vi "FindColllisionPoints.vi"(6 "enemy_robots":T1[](array[typedef]), 7 "our_robots":T1[](array[typedef]), 8 "Robot in":T1, 9 "Goal":dbl[](array[numeric]), 10 "Initial State":dbl[](array[numeric]), 11 "ball":dbl[](array[numeric])) -> (2 "Collision Points":dbl[][](array[numeric]))   [LabVIEW 2017]
uses:
  Core/AI Robot.ctl
  Intel/Functions Enum.ctl
  Intel/AttackerStates.ctl
  PathDests.ctl
  PathDest.ctl
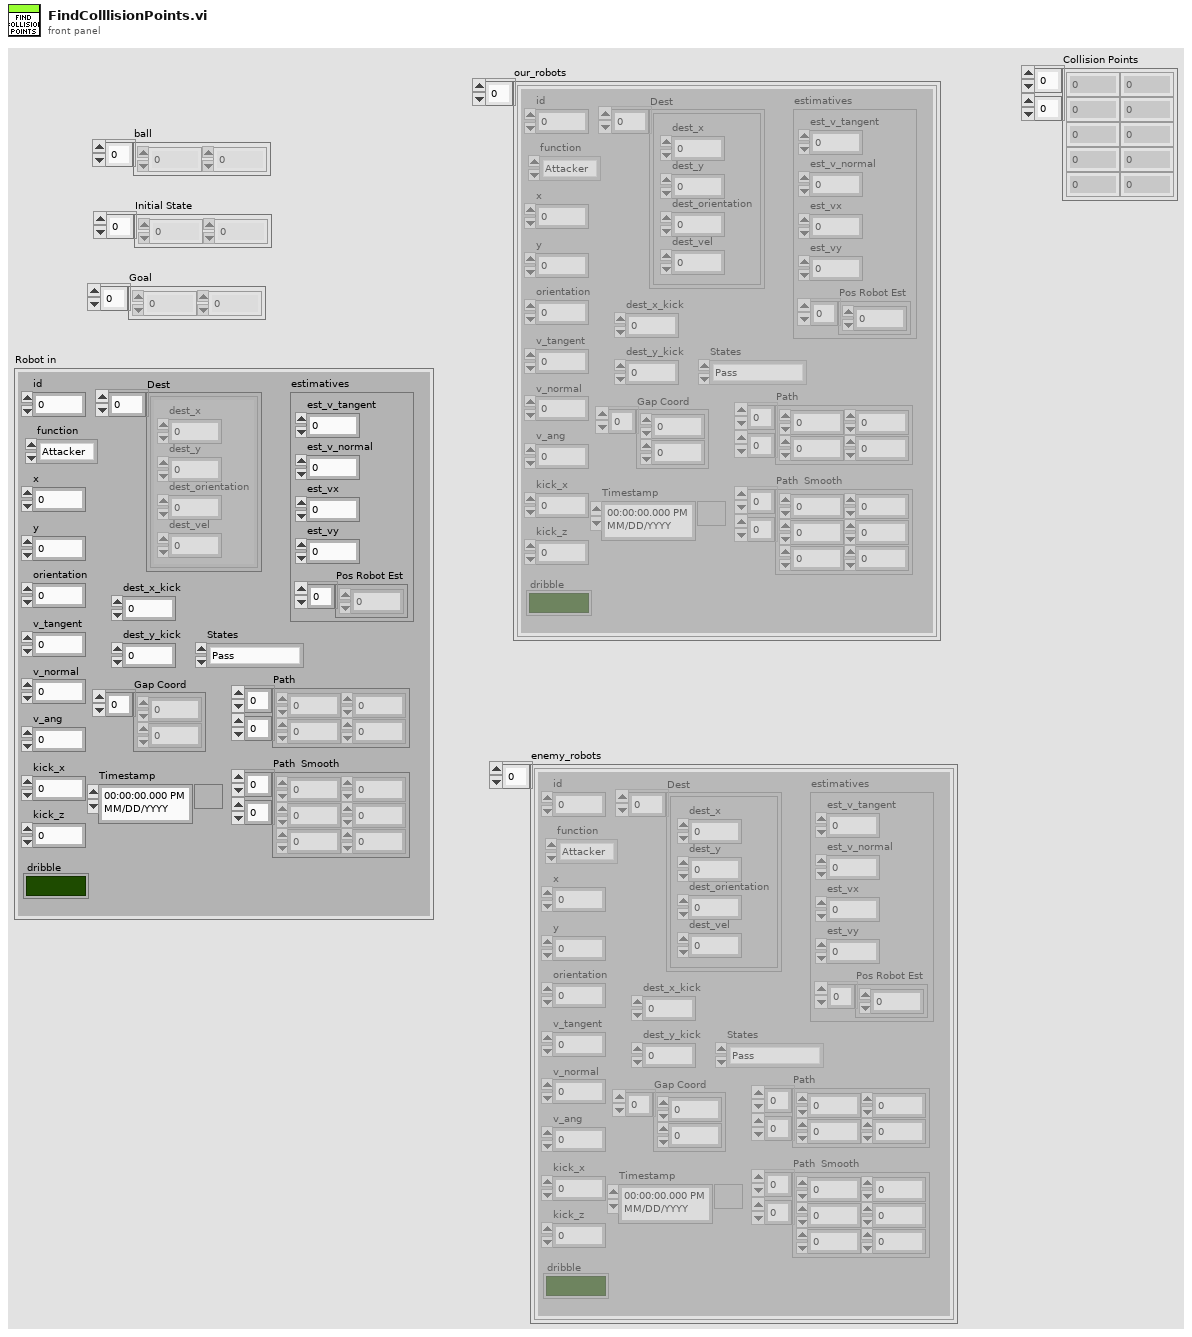
[diagram p1: front panel]
types:
  T1 = typedef "AI Robot.ctl" = cluster{"id":u32, "function":T2, "x":dbl, "y":dbl, "orientation":dbl, "v_tangent":dbl, "v_normal":dbl, "v_ang":dbl, "kick_x":dbl, "kick_z":dbl, "dribble":bool, "Timestamp":timestamp, "estimatives":cluster{"est_v_tangent":dbl, "est_v_normal":dbl, "est_vx":dbl, "est_vy":dbl, "Pos Robot Est":dbl[]}, "dest_x_kick":dbl, "dest_y_kick":dbl, "Gap Coord":dbl[], "States":T3, "Path ":dbl[][], "Path  Smooth":dbl[][], "Dest":T4}
  T2 = typedef "Functions Enum.ctl" = enum16{"Attacker", "Goalie", "Defender", "Striker", "Goto 0", "Dummy", "Kicker", "ZigZag 0", "ZigZag 1", "ZigZag 2", "ZigZag 3", "ZigZag 4", "ZigZag 5", "ZigZag 6", "ZigZag 7", "ZigZag 8", ""}
  T3 = typedef "AttackerStates.ctl" = enum16{"Pass", "GoToTangent", "BallGetting", "GoToKick", ""}
  T4 = typedef "PathDests.ctl" = T5[]
  T5 = typedef "PathDest.ctl" = cluster{"dest_x":dbl, "dest_y":dbl, "dest_orientation":dbl, "dest_vel":dbl}
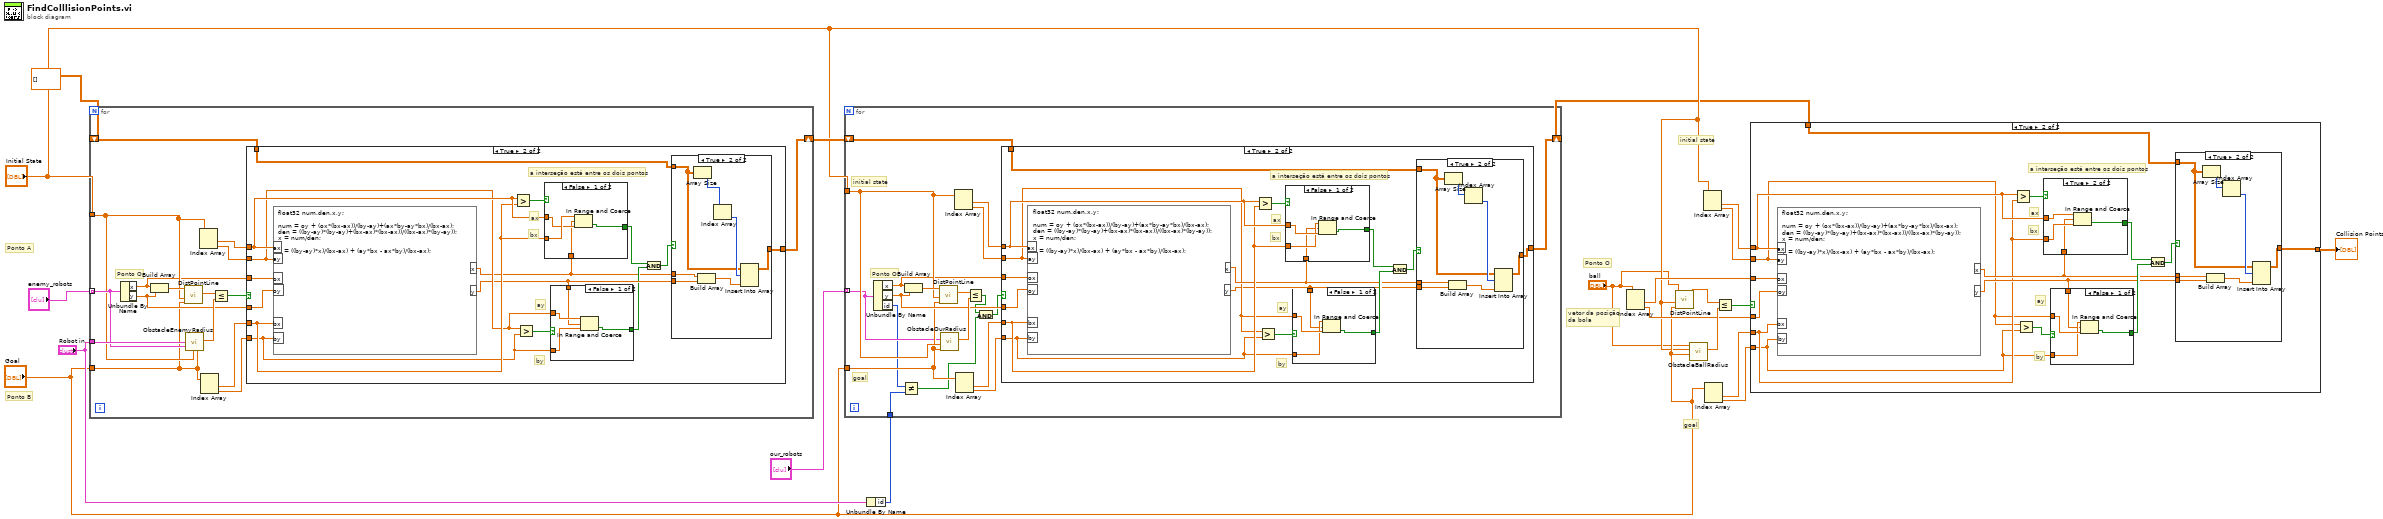
[diagram p0: block diagram]
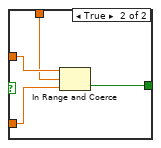
[diagram p4: hidden frame]
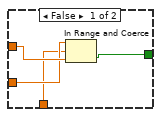
[diagram p5: hidden frame]
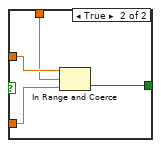
[diagram p8: hidden frame]
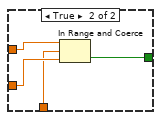
[diagram p9: hidden frame]
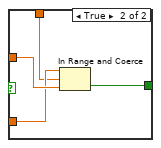
[diagram p12: hidden frame]
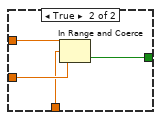
[diagram p13: hidden frame]
diagram:
  # "goal"
  # "initial state"
  # "Ponto O"
  # "vetor da posição\nda bola"
  # "Ponto B"
  # "Ponto A"
  n1 = for {
    tunnel: "enemy_robots" -> [w32] mode=indexing
    tunnel: "Initial State" -> [w28]
    tunnel: "Goal" -> [w23]
    tunnel: "Robot in" -> [w33]
    shift-right: [w29] -> w18
    shift-left: dbl[][] [] ("Path") -> [w30]
    # "Ponto O"
    n2 = Unbundle By Name(w32) -> ("x"=w25:dbl, "y"=w24:dbl)
    n3 = Build Array(w25, w24) -> (w36:dbl[])
    n4 = call "DistPointLine.vi"("P2"=w23, "P1"=w28, "Q"=w36) -> ("distance"=w35:dbl)  [unwired: 8 in]
    n5 = call "ObstacleEnemyRadius.vi"("Goal"=w23, "Initial State"=w28, "Robot enemy"=w32, "Robot in"=w33) -> ("obstacle enemy radius"=w34:dbl)  [unwired: 7 in]
    n6 = Index Array(array=w28) -> (element #1=w27:dbl, element #2=w26:dbl)  [unwired: 2 in]
    n7 = Index Array(array=w23) -> (element #1=w22:dbl, element #2=w21:dbl)  [unwired: 2 in]
    n8 = Less Or Equal?(x=w35, y=w34) -> (x <= y?=w31:bool)
    n9 = case shown="True" w31 {
      tunnel: w30 -> [w37 w50]
      tunnel: [w37 w49] -> w29
      tunnel: w27 -> [_ w47]
      tunnel: w26 -> [_ w44]
      tunnel: w25 -> [_ w52]
      tunnel: w24 -> [_ w51]
      tunnel: w22 -> [_ w46]
      tunnel: w21 -> [_ w43]
      frame False {
        # "obstáculo longe da trajetória"
      }
      frame True {
        # "a interseção está entre os dois pontos"
        # "by"
        # "ay"
        # "bx"
        # "ax"
        n10 = formula code="float32 num,den,x,y;\n\nnum = oy + (ox*(bx-ax))/(by-ay)+(ax*by-ay*bx)/(bx-ax);\nden = ((by-ay)*(by-ay)+(bx-ax)*(bx-ax))/((bx-ax)*(by-ay));\nx = num/den;\n\ny = ((by-ay)*x)/(bx-ax) + (ay*bx - ax*by)/(bx-ax);"("ax"=w47, "ay"=w44, "ox"=w52, "oy"=w51, "bx"=w46, "by"=w43) -> ("x"=w39:sgl, "y"=w42:sgl)
        n11 = Greater?(x=w47, y=w46) -> (0:w48:bool)
        n12 = Greater?(x=w44, y=w43) -> (0:w45:bool)
        n13 = case shown="False" w48 {
          tunnel: w47 -> [w71 w76]
          tunnel: w46 -> [w72 w75]
          tunnel: [w70 w74] -> w41
          tunnel: w39 -> [w69 w73]
          frame False {
            n14 = In Range and Coerce(upper limit=w72, x=w69, lower limit=w71) -> (In Range?=w70:bool)  [unwired: 1 out]
          }
          frame True {
            n15 = In Range and Coerce(upper limit=w76, x=w73, lower limit=w75) -> (In Range?=w74:bool)  [unwired: 1 out]
          }
        }
        n16 = case shown="False" w45 {
          tunnel: [w64 w68] -> w40
          tunnel: w44 -> [w63 w67]
          tunnel: w43 -> [w62 w66]
          tunnel: w42 -> [w61 w65]
          frame False {
            n17 = In Range and Coerce(upper limit=w63, x=w61, lower limit=w62) -> (In Range?=w64:bool)  [unwired: 1 out]
          }
          frame True {
            n18 = In Range and Coerce(upper limit=w66, x=w65, lower limit=w67) -> (In Range?=w68:bool)  [unwired: 1 out]
          }
        }
        n19 = And(x=w41, y=w40) -> (x .and. y?=w38:bool)
        n20 = case shown="True" w38 {
          tunnel: w50 -> [w53 w57]
          tunnel: [w53 w56] -> w49
          tunnel: w42 -> [_ w55]
          tunnel: w39 -> [_ w54]
          frame False {
          }
          frame True {
            n21 = Array Size(array=w57) -> (size(s)=w60:i32[])
            n22 = Build Array(w54, w55) -> (w58:sgl[])
            n23 = Index Array(array=w60) -> (element=w59:i32)  [unwired: 1 in]
            n24 = Insert Into Array(array=w57, index (row)=w59, new element=w58) -> (w56:dbl[][])  [unwired: 1 in]
          }
        }
      }
    }
  }
  n25 = Unbundle By Name("Robot in") -> ("id"=w15:u32)
  n26 = for {
    tunnel: "our_robots" -> [w82] mode=indexing
    tunnel: "Initial State" -> [w90]
    tunnel: "Goal" -> [w85]
    shift-right: [w91] -> w2
    shift-left: w18 -> [w92]
    tunnel: w15 -> [w81]
    # "goal"
    # "initial state"
    # "Ponto O"
    n27 = Unbundle By Name(w82) -> ("x"=w87:dbl, "y"=w86:dbl, "id"=w80:u32)
    n28 = Not Equal?(x=w80, y=w81) -> (x != y?=w78:bool)
    n29 = Build Array(w87, w86) -> (w95:dbl[])
    n30 = call "DistPointLine.vi"("P2"=w85, "P1"=w90, "Q"=w95) -> ("distance"=w94:dbl)  [unwired: 8 in]
    n31 = call "ObstacleOurRadius.vi"("Goal"=w85, "Initial State"=w90, "other robot"=w82) -> ("obstacle enemy radius"=w93:dbl)  [unwired: 8 in]
    n32 = Index Array(array=w90) -> (element #1=w89:dbl, element #2=w88:dbl)  [unwired: 2 in]
    n33 = Index Array(array=w85) -> (element #1=w84:dbl, element #2=w83:dbl)  [unwired: 2 in]
    n34 = Less Or Equal?(x=w94, y=w93) -> (x <= y?=w79:bool)
    n35 = And(x=w79, y=w78) -> (x .and. y?=w77:bool)
    n36 = case shown="True" w77 {
      tunnel: w92 -> [w96 w109]
      tunnel: [w96 w108] -> w91
      tunnel: w89 -> [_ w103]
      tunnel: w88 -> [_ w100]
      tunnel: w87 -> [_ w111]
      tunnel: w86 -> [_ w110]
      tunnel: w84 -> [_ w102]
      tunnel: w83 -> [_ w99]
      frame False {
        # "obstáculo longe da trajetória"
      }
      frame True {
        # "a interseção está entre os dois pontos"
        # "by"
        # "ay"
        # "bx"
        # "ax"
        n37 = formula code="float32 num,den,x,y;\n\nnum = oy + (ox*(bx-ax))/(by-ay)+(ax*by-ay*bx)/(bx-ax);\nden = ((by-ay)*(by-ay)+(bx-ax)*(bx-ax))/((bx-ax)*(by-ay));\nx = num/den;\n\ny = ((by-ay)*x)/(bx-ax) + (ay*bx - ax*by)/(bx-ax);"("ax"=w103, "ay"=w100, "ox"=w111, "oy"=w110, "bx"=w102, "by"=w99) -> ("x"=w101:sgl, "y"=w98:sgl)
        n38 = Greater?(x=w103, y=w102) -> (0:w107:bool)
        n39 = Greater?(x=w100, y=w99) -> (0:w106:bool)
        n40 = case shown="False" w107 {
          tunnel: [w131 w135] -> w105
          tunnel: w103 -> [w130 w134]
          tunnel: w102 -> [w129 w133]
          tunnel: w101 -> [w128 w132]
          frame False {
            n41 = In Range and Coerce(upper limit=w129, x=w128, lower limit=w130) -> (In Range?=w131:bool)  [unwired: 1 out]
          }
          frame True {
            n42 = In Range and Coerce(upper limit=w134, x=w132, lower limit=w133) -> (In Range?=w135:bool)  [unwired: 1 out]
          }
        }
        n43 = case shown="False" w106 {
          tunnel: [w123 w127] -> w104
          tunnel: w100 -> [w122 w126]
          tunnel: w99 -> [w121 w125]
          tunnel: w98 -> [w120 w124]
          frame False {
            n44 = In Range and Coerce(upper limit=w121, x=w120, lower limit=w122) -> (In Range?=w123:bool)  [unwired: 1 out]
          }
          frame True {
            n45 = In Range and Coerce(upper limit=w126, x=w124, lower limit=w125) -> (In Range?=w127:bool)  [unwired: 1 out]
          }
        }
        n46 = And(x=w105, y=w104) -> (x .and. y?=w97:bool)
        n47 = case shown="True" w97 {
          tunnel: w109 -> [w112 w116]
          tunnel: [w112 w115] -> w108
          tunnel: w101 -> [_ w114]
          tunnel: w98 -> [_ w113]
          frame False {
          }
          frame True {
            n48 = Array Size(array=w116) -> (size(s)=w119:i32[])
            n49 = Build Array(w114, w113) -> (w117:sgl[])
            n50 = Index Array(array=w119) -> (element=w118:i32)  [unwired: 1 in]
            n51 = Insert Into Array(array=w116, index (row)=w118, new element=w117) -> (w115:dbl[][])  [unwired: 1 in]
          }
        }
      }
    }
  }
  n52 = Index Array(array="ball") -> (element #1=w7:dbl, element #2=w6:dbl)  [unwired: 2 in]
  n53 = call "DistPointLine.vi"("P2"="Goal", "P1"="Initial State", "Q"="ball") -> ("distance"=w14:dbl)  [unwired: 8 in]
  n54 = call "ObstacleBallRadius.vi"("Goal"="Goal", "Initial State"="Initial State", "ball"="ball") -> ("obstacle enemy radius"=w13:dbl)  [unwired: 8 in]
  n55 = Index Array(array="Initial State") -> (element #1=w11:dbl, element #2=w10:dbl)  [unwired: 2 in]
  n56 = Index Array(array="Goal") -> (element #1=w9:dbl, element #2=w8:dbl)  [unwired: 2 in]
  n57 = Less Or Equal?(x=w14, y=w13) -> (x <= y?=w12:bool)
  n58 = case shown="True" w12 {
    tunnel: [w136 w141] -> w1
    tunnel: w11 -> [_ w140]
    tunnel: w10 -> [_ w137]
    tunnel: w7 -> [_ w151]
    tunnel: w6 -> [_ w150]
    tunnel: w9 -> [_ w139]
    tunnel: w8 -> [_ w138]
    tunnel: w2 -> [w136 w142]
    frame False {
      # "obstáculo longe da trajetória"
    }
    frame True {
      # "a interseção está entre os dois pontos"
      # "by"
      # "ay"
      # "bx"
      # "ax"
      n59 = formula code="float32 num,den,x,y;\n\nnum = oy + (ox*(bx-ax))/(by-ay)+(ax*by-ay*bx)/(bx-ax);\nden = ((by-ay)*(by-ay)+(bx-ax)*(bx-ax))/((bx-ax)*(by-ay));\nx = num/den;\n\ny = ((by-ay)*x)/(bx-ax) + (ay*bx - ax*by)/(bx-ax);"("ax"=w140, "ay"=w137, "ox"=w151, "oy"=w150, "bx"=w139, "by"=w138) -> ("x"=w144:sgl, "y"=w143:sgl)
      n60 = Greater?(x=w140, y=w139) -> (0:w149:bool)
      n61 = Greater?(x=w137, y=w138) -> (0:w148:bool)
      n62 = case shown="True" w149 {
        tunnel: [w171 w175] -> w147
        tunnel: w140 -> [w170 w174]
        tunnel: w139 -> [w169 w173]
        tunnel: w144 -> [w168 w172]
        frame False {
          n63 = In Range and Coerce(upper limit=w169, x=w168, lower limit=w170) -> (In Range?=w171:bool)  [unwired: 1 out]
        }
        frame True {
          n64 = In Range and Coerce(upper limit=w174, x=w172, lower limit=w173) -> (In Range?=w175:bool)  [unwired: 1 out]
        }
      }
      n65 = case shown="False" w148 {
        tunnel: [w163 w167] -> w146
        tunnel: w137 -> [w162 w166]
        tunnel: w138 -> [w161 w165]
        tunnel: w143 -> [w160 w164]
        frame False {
          n66 = In Range and Coerce(upper limit=w161, x=w160, lower limit=w162) -> (In Range?=w163:bool)  [unwired: 1 out]
        }
        frame True {
          n67 = In Range and Coerce(upper limit=w166, x=w164, lower limit=w165) -> (In Range?=w167:bool)  [unwired: 1 out]
        }
      }
      n68 = And(x=w147, y=w146) -> (x .and. y?=w145:bool)
      n69 = case shown="True" w145 {
        tunnel: w142 -> [w152 w156]
        tunnel: [w152 w155] -> w141
        tunnel: w144 -> [_ w154]
        tunnel: w143 -> [_ w153]
        frame False {
        }
        frame True {
          n70 = Array Size(array=w156) -> (size(s)=w159:i32[])
          n71 = Build Array(w154, w153) -> (w157:sgl[])
          n72 = Index Array(array=w159) -> (element=w158:i32)  [unwired: 1 in]
          n73 = Insert Into Array(array=w156, index (row)=w158, new element=w157) -> (w155:dbl[][])  [unwired: 1 in]
        }
      }
    }
  }
  "Collision Points" <- w1
